vi "Launch Sub Loop.vi"(4 "Bind Address":string, 6 "DataHandler":refnum<class "SubscribedDataHandler.lvclass">, 7 "Telemetry Config":T1, 9 "Subscription Info":T5, 10 "Subscription":T4, 11 "ChannelService":refnum<class "ChannelService.lvclass">) -> (0 "error out":errorcluster)   [LabVIEW 2020, in "Vecto.lvlib" / "RemoteDataService.lvclass"]
uses:
  RemoteDataService.lvclass
  Subscription Info.ctl
  SubscribedDataHandler/SubscribedDataHandler.lvclass
  Subscription.ctl
  ChannelService/ChannelService.lvclass
  lv-promises/Promises/Error Result/Error Result.lvclass
  lv-promises/Promises/Promise/Promise.lvclass/Promise.ctl
  lv-promises/Promises/Future/Future.lvclass/Future.ctl
  lv-promises/Promises/Error Result/Error Result.lvclass/Error Result.ctl
  Subscription Loop.vi
  lv-promises/Promises/Future/Future.lvclass
  RemoteDataService.lvclass/RemoteDataService.ctl
  lv-promises/Promises/Promise/Promise.lvclass
  VectoConfig/Telemetry Routing.ctl
  VectoConfig/VectoConfig.lvlib
  VectoConfig/Endpoint.ctl
  VectoConfig/Telemetry Config.ctl
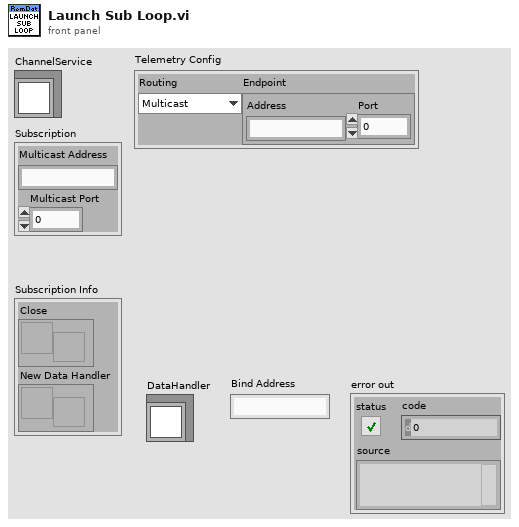
[diagram p1: front panel]
types:
  T1 = typedef "VectoConfig.lvlib/Telemetry Config.ctl" = cluster{"Routing":T2, "Endpoint":T3}
  T2 = typedef "VectoConfig.lvlib/Telemetry Routing.ctl" = enum16{"Multicast", "Unicast"}
  T3 = typedef "VectoConfig.lvlib/Endpoint.ctl" = cluster{"Address":string, "Port":u16}
  T4 = typedef "Vecto.lvlib/RemoteDataService.lvclass/Subscription.ctl" = cluster{"Multicast Address":string, "Multicast Port":u16}
  T5 = typedef "Vecto.lvlib/RemoteDataService.lvclass/Subscription Info.ctl" = cluster{"Close":refnum<user-event>, "New Data Handler":refnum<user-event>}
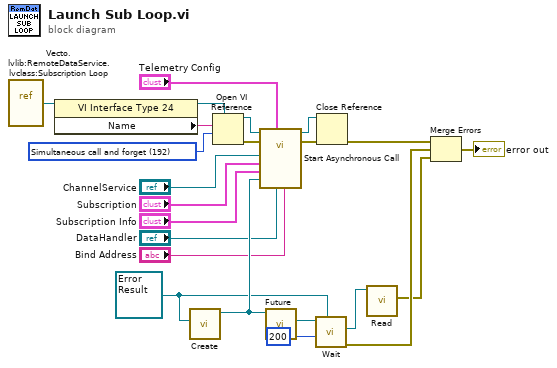
[diagram p0: block diagram]
diagram:
  w10 = refnum<class "Error Result.lvclass"> refnum ("Futures:Error Result.lvclass")
  w18 = 192 items=["Record modifications"=1, "Open templates for editing"=2, "Prompt user to save"=4, "Prepare for reentrant run"=8, "Prompt to find missing subVIs"=16, "Hide loading dialog box"=32, "Enable simultaneous calls"=64, "Prepare to call and forget"=128, "Simultaneous call and forget"=192, "Prepare to call and collect"=256, "Simultaneous call and collect"=320]
  n1 = vi-ref "Vecto.lvlib:RemoteDataService.lvclass:Subscription Loop.vi"() -> (w16:refnum<vi>)
  n2 = property class="VI Interface Type 24"(reference=w16) -> (reference out=w19:refnum<vi>, "Name"=w17:string)  [unwired: 1 in, 1 out]
  n3 = call "Create.vi"("Result Type (None)"=w10) -> ("Promise"=w12:refnum<class "Promise.lvclass">)  [unwired: 9 in, 1 out]
  n4 = Open VI Reference(type specifier VI Refnum (for type only)=w19, vi path=w17, options=w18) -> (vi reference=w21:refnum<vi>, error out=w20:errorcluster)  [unwired: 3 in]
  n5 = call-by-ref "Start Asynchronous Call"(reference=w21, error in=w20, "Bind Address"="Bind Address", "DataHandler"="DataHandler", "Telemetry Config"="Telemetry Config", "Init Promise"=w12, "Subscription Info"="Subscription Info", "Subscription"="Subscription", "ChannelService"="ChannelService") -> (reference out=w23:refnum<vi>, error out=w22:errorcluster)  [unwired: 5 in]
  n6 = call "Future.vi"("Promise in"=w12) -> ("Future"=w11:refnum<class "Future.lvclass">)  [unwired: 9 in, 1 out]
  n7 = call "Wait.vi"("Result Type (None)"=w10, "Timeout mS (-1)"=200, "Future in"=w11) -> ("error out"=w6:errorcluster, "Result"=w9:refnum<class "Error Result.lvclass">)  [unwired: 7 in]
  n8 = Close Reference(reference=w23, error in (no error)=w22) -> (error out=w8:errorcluster)
  n9 = call "Read.vi"("Error Result in"=w9) -> ("Error"=w5:errorcluster)  [unwired: 10 in]
  n10 = Merge Errors(w8, w6, w5) -> (→"error out":errorcluster)
